vi "Math-Uniform Random Number (DBL, scalar).vi"(4 "Ymax":dbl, 5 "Ymin":dbl) -> (1 "Random Value":dbl)   [LabVIEW 2020]
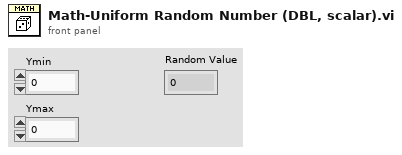
[diagram p1: front panel]
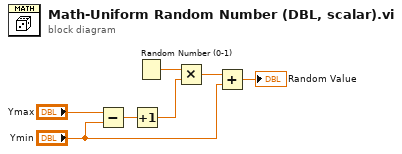
[diagram p0: block diagram]
diagram:
  n1 = Subtract(x="Ymax", y="Ymin") -> (x-y=w6:dbl)
  n2 = Increment(x=w6) -> (x+1=w5:dbl)
  n3 = Random Number (0-1)() -> (number: 0 to 1=w7:dbl)
  n4 = Multiply(x=w7, y=w5) -> (x*y=w1:dbl)
  n5 = Add(x=w1, y="Ymin") -> (x+y=→"Random Value":dbl)
